vi "Timing_Tests.vi"() -> ()   [LabVIEW 2014]
uses:
  <vilib>/Utility/miscctls.llb/LVDateTimeRec.ctl
panel:
  out "date time rec":T1
  out "current time":timestamp
  out "millisecond timer value":u32
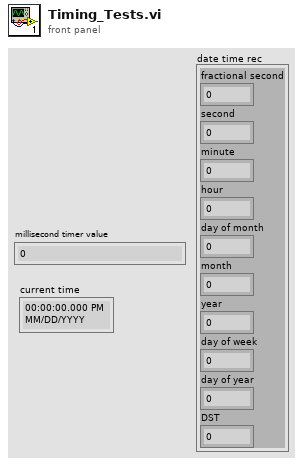
[diagram p1: front panel]
types:
  T1 = typedef "LVDateTimeRec.ctl" = cluster{"fractional second":dbl, "second":i32, "minute":i32, "hour":i32, "day of month":i32, "month":i32, "year":i32, "day of week":i32, "day of year":i32, "DST":i32}
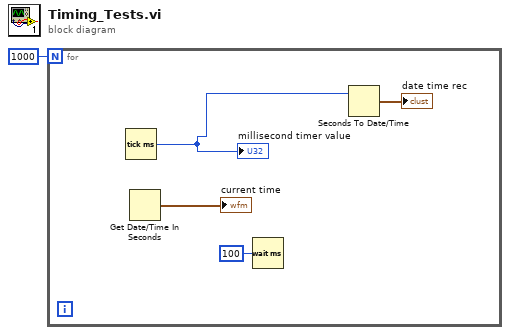
[diagram p0: block diagram]
diagram:
  n1 = for {
    N: 1000 -> [_]
    n2 = Tick Count (ms)() -> (millisecond timer value=w3:u32)
    "millisecond timer value" <- w3
    n3 = Get Date/Time In Seconds() -> (seconds since 1Jan1904=→"current time":timestamp)
    n4 = Wait (ms)(milliseconds to wait=u32 100) -> ()  [unwired: 1 out]
    n5 = Seconds To Date/Time(time stamp (now)=w3) -> (date time rec=→"date time rec":T1)  [unwired: 1 in]
  }
